vi "makeDirectoryIfRequired.vi"(8 "error in (no error)":errorcluster, 11 "BaseSetting in":refnum<class "Setting.lvclass">) -> (0 "error out":errorcluster, 3 "BaseSetting out":refnum<class "Setting.lvclass">)   [LabVIEW 2016, in "Setting.lvclass"]
uses:
  Setting.lvclass
  Setting.lvclass/Setting.ctl
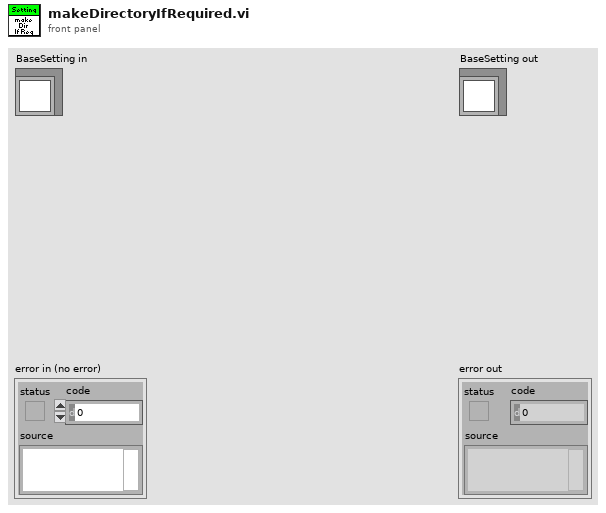
[diagram p1: front panel]
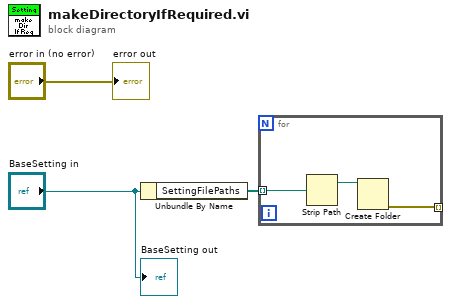
[diagram p0: block diagram]
diagram:
  n1 = Unbundle By Name("BaseSetting in") -> ("SettingFilePaths"=w3:path[])
  n2 = for {
    tunnel: w3 -> [w6] mode=indexing
    tunnel: [w4] -> _ mode=indexing
    n3 = Strip Path(path=w6) -> (stripped path=w5:path)  [unwired: 1 out]
    n4 = Create Folder(path (use dialog)=w5) -> (error out=w4:errorcluster)  [unwired: 2 in, 2 out]
  }
  "error out" <- "error in (no error)"
  "BaseSetting out" <- "BaseSetting in"
